vi "caxis_best_fit_for_trials.vi"(8 "Error In":errorcluster, 9 "phic":dbl[](array[numeric]), 10 "thetac":dbl[](array[numeric]), 11 "Sample Results":T1) -> (0 "Error Out":errorcluster, 1 "Best R2":dbl[](array[numeric]), 2 "Theta min":dbl[](array[numeric]), 3 "Phi min":dbl[](array[numeric]))   [LabVIEW 2019]
uses:
  sample_results_cluster_typedef.ctl
  parameters_cluster_typedef.ctl
  writeable_section_parameters_cluster_typedef.ctl
  grain_results_cluster_typedef.ctl
  xtal_description_for_prediction_cluster_typedef.ctl
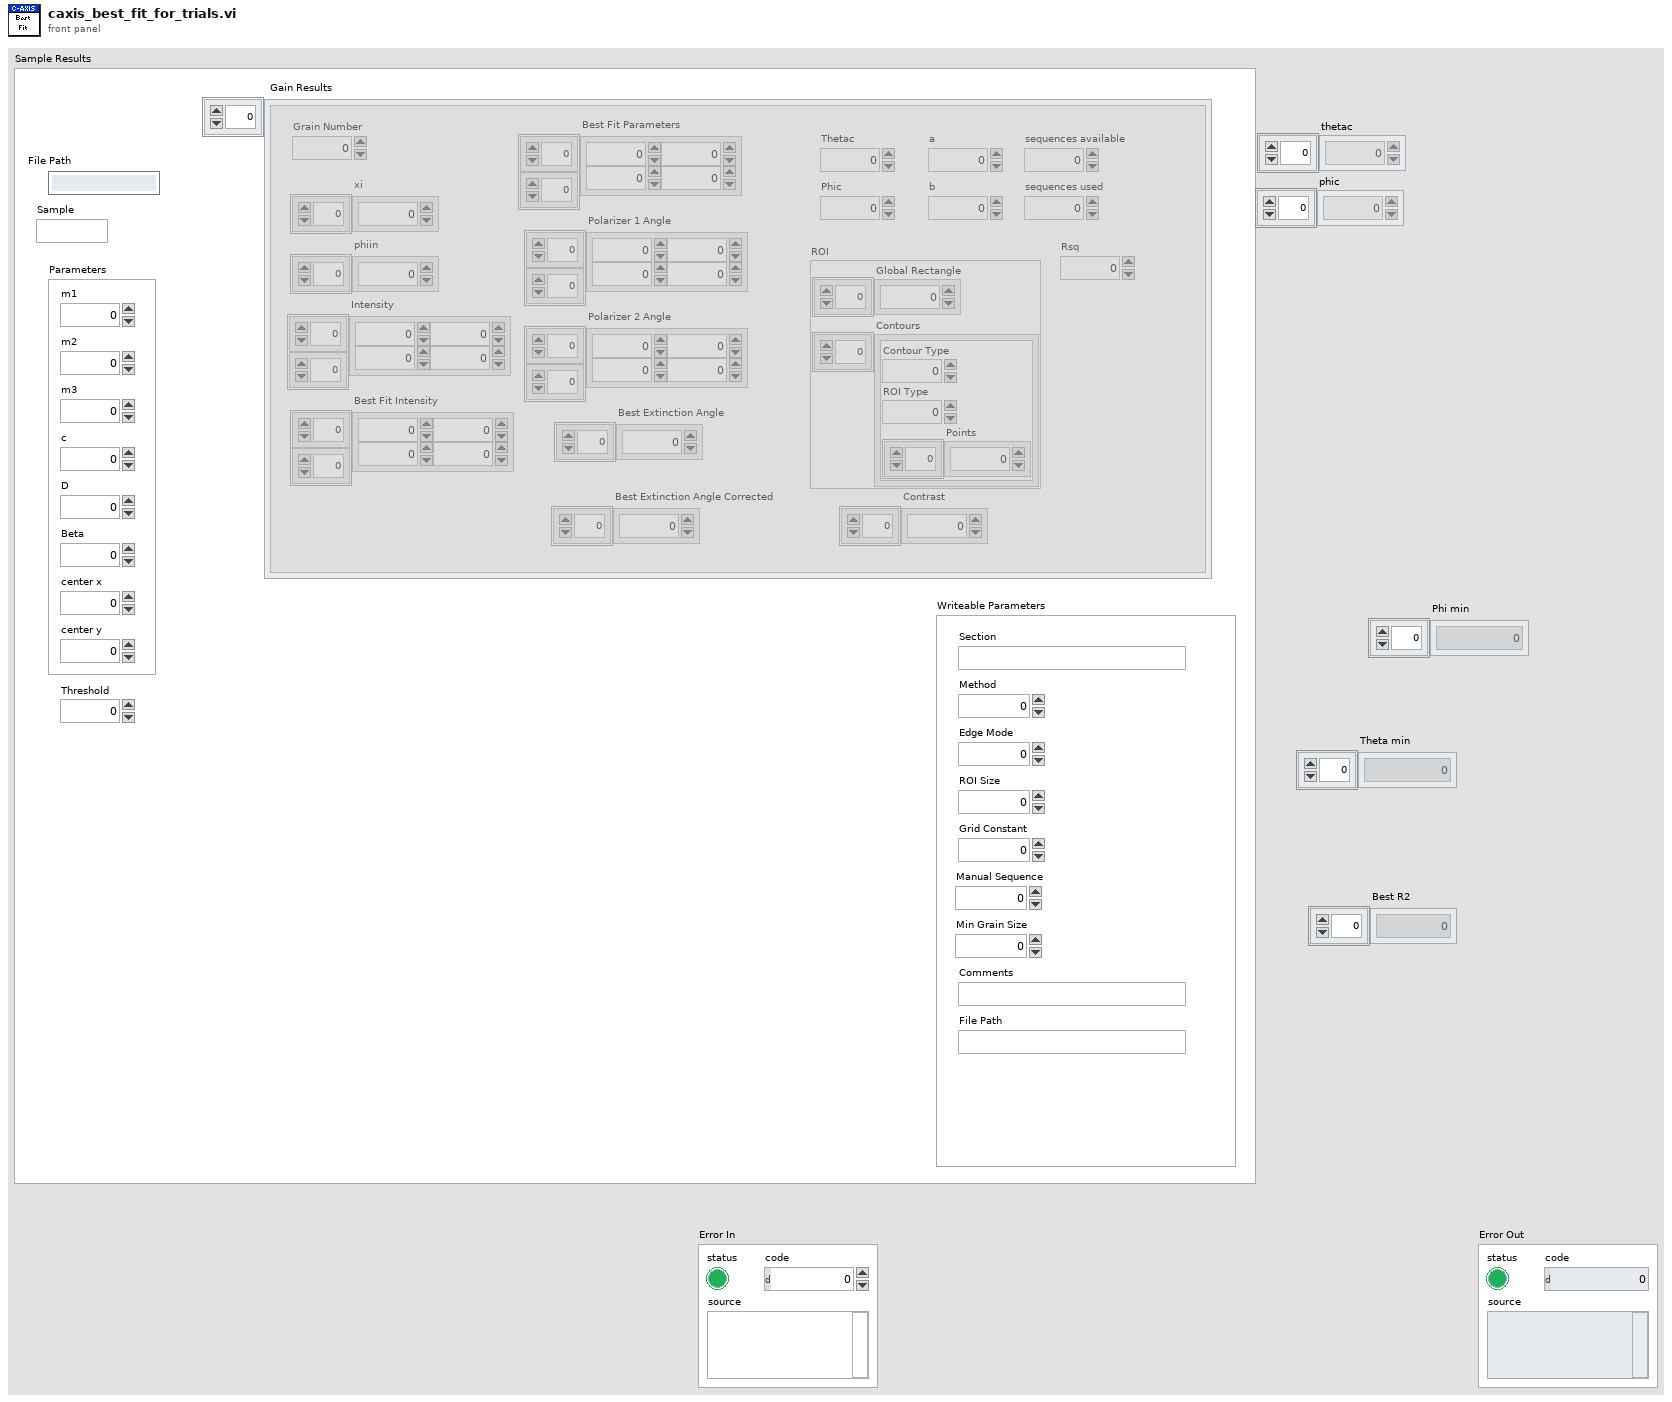
[diagram p1: front panel]
types:
  T1 = typedef "sample_results_cluster_typedef.ctl" = cluster{"File Path":string, "Sample":string, "Threshold":dbl, "Parameters":T2, "Writeable Parameters":T3, "Gain Results":T4[]}
  T2 = typedef "parameters_cluster_typedef.ctl" = cluster{"m1":dbl, "m2":dbl, "m3":dbl, "c":dbl, "D":dbl, "Beta":dbl, "center x":dbl, "center y":dbl}
  T3 = typedef "writeable_section_parameters_cluster_typedef.ctl" = cluster{"Section":string, "Method":i32, "Edge Mode":i32, "Grid Constant":i32, "Manual Sequence":i32, "ROI Size":i32, "Min Grain Size":dbl, "Comments":string, "File Path":string}
  T4 = typedef "grain_results_cluster_typedef.ctl" = cluster{"Grain Number":i32, "xi":dbl[], "phiin":dbl[], "Intensity":dbl[][], "Best Fit Intensity":dbl[][], "Best Fit Parameters":dbl[][], "Polarizer 1 Angle":dbl[][], "Polarizer 2 Angle":dbl[][], "Best Extinction Angle":dbl[], "Best Extinction Angle Corrected":dbl[], "Thetac":dbl, "Phic":dbl, "ROI":cluster{"Global Rectangle":i32[], "Contours":cluster{"Contour Type":u32, "ROI Type":u32, "Points":i32[]}[]}, "a":dbl, "b":dbl, "sequences available":dbl, "sequences used":dbl, "Contrast":dbl[], "Rsq":dbl}
  T5 = typedef "xtal_description_for_prediction_cluster_typedef.ctl" = cluster{"xi":dbl, "phi in":dbl, "phi c":dbl, "theta c":dbl, "m3":dbl, "a":dbl, "b":dbl, "c":dbl, "D":dbl}
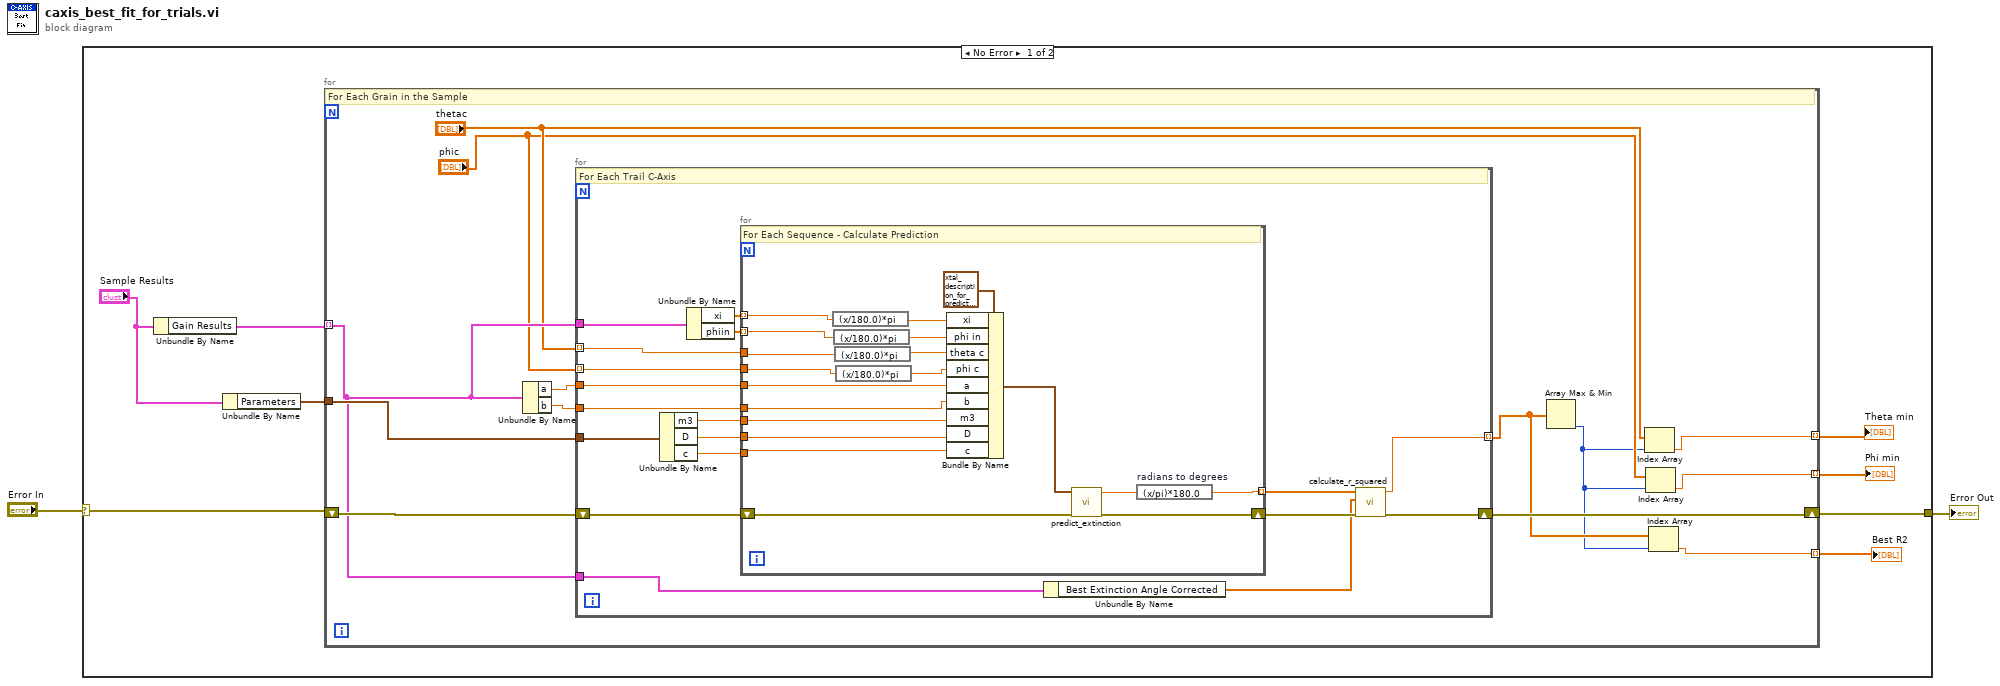
[diagram p0: block diagram]
diagram:
  n1 = case shown="No Error" "Error In" {
    selector: "Error In" -> [w7 w61]
    tunnel: [w6 w61] -> w1
    frame No Error {
      n2 = Unbundle By Name("Sample Results") -> ("Gain Results"=w8:T4[])
      n3 = Unbundle By Name("Sample Results") -> ("Parameters"=w9:T2)
      n4 = for {
        tunnel: w8 -> [w19] mode=indexing
        shift-right: [w18] -> w6
        shift-left: w7 -> [w23]
        tunnel: w9 -> [w22]
        tunnel: [w13] -> w4 mode=indexing
        tunnel: [w12] -> w5 mode=indexing
        tunnel: [w11] -> w3 mode=indexing
        # "For Each Grain in the Sample"
        n5 = Unbundle By Name(w19) -> ("a"=w21:dbl, "b"=w20:dbl)
        n6 = for {
          shift-right: [w28] -> w18
          shift-left: w23 -> [w41]
          tunnel: w22 -> [w40]
          tunnel: w19 -> [w29]
          tunnel: "phic" -> [w36] mode=indexing
          tunnel: "thetac" -> [w35] mode=indexing
          tunnel: w21 -> [w34]
          tunnel: w20 -> [w33]
          tunnel: w19 -> [w32]
          tunnel: [w24] -> w15 mode=indexing
          # "For Each Trail C-Axis"
          n7 = Unbundle By Name(w40) -> ("m3"=w39:dbl, "D"=w38:dbl, "c"=w37:dbl)
          n8 = Unbundle By Name(w32) -> ("xi"=w31:dbl[], "phiin"=w30:dbl[])
          n9 = for {
            shift-right: [w57] -> w27
            shift-left: w41 -> [w58]
            tunnel: w35 -> [w45]
            tunnel: w36 -> [w44]
            tunnel: w39 -> [w56]
            tunnel: w38 -> [w55]
            tunnel: w37 -> [w54]
            tunnel: [w43] -> w26 mode=indexing
            tunnel: w34 -> [w53]
            tunnel: w33 -> [w52]
            tunnel: w31 -> [w47] mode=indexing
            tunnel: w30 -> [w46] mode=indexing
            # "For Each Sequence - Calculate Prediction"
            n10 = expression code="(x/180.0)*pi" ("degrees to radians")(w47) -> (w48:dbl)
            n11 = expression code="(x/180.0)*pi" ("degrees to radians")(w46) -> (w49:dbl)
            n12 = expression code="(x/180.0)*pi" ("degrees to radians")(w45) -> (w50:dbl)
            n13 = expression code="(x/180.0)*pi" ("degrees to radians")(w44) -> (w51:dbl)
            n14 = Bundle By Name(cluster=T5 {"xi"=0.0, "phi in"=0.0, "phi c"=0.0, "theta c"=0.0, "m3"=0.0, "a"=0.0, "b"=0.0, "c"=0.0, "D"=0.0} ("Xtal Description"), "xi"=w48, "phi in"=w49, "theta c"=w50, "phi c"=w51, "a"=w53, "b"=w52, "m3"=w56, "D"=w55, "c"=w54) -> (w59:T5)
            n15 = call "predict_extinction.vi"("Error In"=w58, "Xtal Description"=w59) -> ("Error Out"=w57:errorcluster, "prediction"=w42:dbl)  [unwired: 8 in]
            n16 = expression code="(x/pi)*180.0" "radians to degrees"(w42) -> (w43:dbl)
          }
          n17 = Unbundle By Name(w29) -> ("Best Extinction Angle Corrected"=w25:dbl[])
          n18 = call "calculate_r_squared.vi"("Error In"=w27, "Expected"=w25, "Fits"=w26) -> ("Error Out"=w28:errorcluster, "R2"=w24:dbl)  [unwired: 7 in]
        }
        n19 = Array Max & Min(array=w15) -> (min index (indices)=w14:i32)  [unwired: 3 out]
        n20 = Index Array(array="thetac", index=w14) -> (element=w13:dbl)
        n21 = Index Array(array="phic", index=w14) -> (element=w12:dbl)
        n22 = Index Array(array=w15, index=w14) -> (element=w11:dbl)
      }
      "Phi min" <- w5
      "Theta min" <- w4
      "Best R2" <- w3
    }
    frame Error {
    }
  }
  "Error Out" <- w1
